vi "updateWaypoints.vi"(8 "error in (no error)":errorcluster, 11 "StationKeeping in":refnum<class "StationKeeping.lvclass">) -> (0 "error out":errorcluster, 3 "StationKeeping out":refnum<class "StationKeeping.lvclass">)   [LabVIEW 2011, in "StationKeeping.lvclass"]
doc: "Handles the 3 phases of the station keeping mission, while it is in progress. Using a timer, it checks which phase of the mission it is in. In the first phase, it calls \"station_keeping_waypoints.vi\" and adds waypoints to the waypoints array from a pattern in that VI. In the second phase, it adds waypoints along the edge of the boundary. In the third phase, it adds a waypoint outside the boundary (w/out a No-Sail Zone)"
uses:
  StationKeeping.lvclass
  StationKeeping.lvclass/StationKeeping.ctl
  2 Globals/2 Global.vi
  Waypoint/Waypoint.lvclass
panel:
  out "Time Elapsed":dbl
  out "Time Remaining":dbl
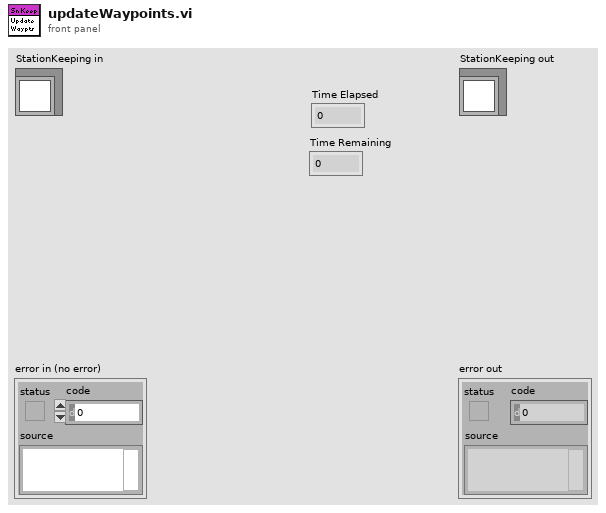
[diagram p1: front panel]
types:
  T1 = typedef "UTM Location.ctl" = cluster{"UTM Zone":dbl, "Hemisphere":enum16{"North", "South"}, "East":dbl, "North":dbl}
  T2 = typedef "UTM Circle.ctl" = cluster{"UTM Zone":dbl, "Hemisphere":enum16{"North", "South"}, "East":dbl, "North":dbl, "Radius":dbl}
  T3 = typedef "Current Waypoint.ctl" = i32
  T4 = typedef "Waypoints List.ctl" = refnum<class "Waypoint.lvclass">[]
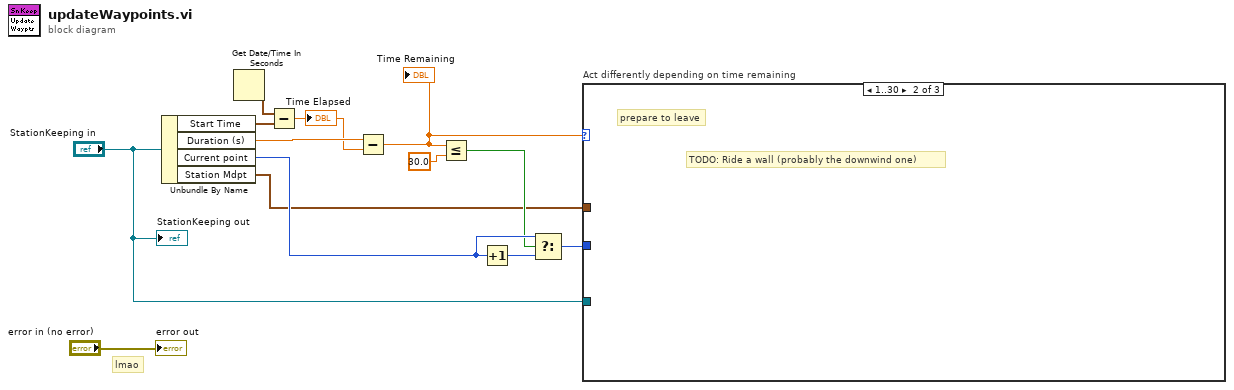
[diagram p0: block diagram]
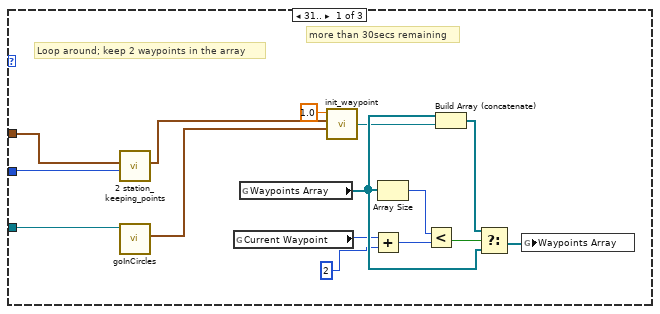
[diagram p2: hidden frame]
diagram:
  # "lmao"
  n1 = Unbundle By Name("StationKeeping in") -> ("Start Time"=w12:timestamp, "Duration (s)"=w11:dbl, "Current point"=w7:i32, "Station Mdpt"=w5:T1)
  n2 = Get Date/Time In Seconds() -> (seconds since 1Jan1904=w13:timestamp)
  n3 = Subtract(x=w13, y=w12) -> (x-y=w10:dbl)
  "Time Elapsed" <- w10
  n4 = Subtract(x=w11, y=w10) -> (x-y=w1:dbl)
  "Time Remaining" <- w1
  n5 = Less Or Equal?(x=w1, y=30.0) -> (x <= y?=w6:bool)
  n6 = Increment(x=w7) -> (x+1=w8:i32)
  n7 = Select(t=w7, s=w6, f=w8) -> (s? t:f=w4:i32)
  n8 = case "Act differently depending on time remaining" shown="1..30" w1 {
    tunnel: w4 -> [w24 _ _]
    tunnel: w5 -> [w18 _ _]
    tunnel: "StationKeeping in" -> [w19 _ _]
    frame 31.. {
      # "more than 30secs remaining"
      # "Loop around; keep 2 waypoints in the array"
      n9 = call "2 station_keeping_points.vi"("Which Point?"=w24, "Midpoint"=w18) -> ("Waypoint"=w23:T1)  [unwired: 9 in]
      n10 = call "goInCircles.vi"("StationKeeping in"=w19) -> ("No Sail Circles"=w17:T2[])  [unwired: 8 in, 2 out]
      n11 = global read "2 Global.vi" "Current Waypoint"() -> (w15:T3)
      n12 = global read "2 Global.vi" "Waypoints Array"() -> (w25:T4)
      n13 = call "init_waypoint.vi"("No Sail Circles"=w17, "Coords"=w23, "Tolerance (m)"=1.0 ("Tolerance (meters?)")) -> ("Waypoint Out"=w22:refnum<class "Waypoint.lvclass">)  [unwired: 8 in]
      n14 = Add(x=w15, y=2) -> (x+y=w14:T3)
      n15 = Array Size(array=w25) -> (size(s)=w28:i32)
      n16 = Less?(x=w28, y=w14) -> (x < y?=w27:bool)
      n17 = Build Array (concatenate)(w25, w22) -> (w26:T4)
      n18 = Select(t=w26, s=w27, f=w25) -> (s? t:f=w21:T4)
      n19 = global write "2 Global.vi" "Waypoints Array"(w21) -> ()
    }
    frame 1..30 {
      # "prepare to leave"
      # "TODO: Ride a wall (probably the downwind one)"
    }
    frame ..0 {
      # "no time remaining"
      # "time has elapsed!"
      # "TODO: Leave the Station"
    }
  }
  "error out" <- "error in (no error)"
  "StationKeeping out" <- "StationKeeping in"
